vi "E710_All_VIs.vi"   [LabVIEW 2011]
uses:
  Low Level/Analog control.llb/Available Analog Commands.ctl
  Low Level/Communication.llb/Available DLL interfaces.ctl
  Low Level/Communication.llb/Available DLLs.ctl
  Low Level/Communication.llb/Available interfaces.ctl
  Low Level/Communication.llb/Termination character.ctl
  Low Level/General command.llb/Controller names.ctl
  Low Level/Analog control.llb/Global Analog.vi
  Low Level/Communication.llb/Global1.vi
  Low Level/Communication.llb/Global DaisyChain.vi
  Low Level/General command.llb/Global2 (Array).vi
  Low Level/Support.llb/Unbunde/bundle interface clusters for PI Terminal.vi
panel:
  # "E-710 PI GCS LabVIEW driver set"
  # "This VI contains all high level and low level VIs valid for E-710. See diagram for a survey of all E-710 high level\nand low level VIs. Menu / Browse / Show VI Hierarchy will show the file paths of the VIs. Global Variables \nare shown as Control as well as Indicator."
types:
  T1 = typedef "Controller names.ctl" = enum16{"None", "Analog", "C-702", "C-843", "C-843.PM", "C-844", "C-848", "C-865", "C-866", "C-867", "C-880", "E-516", "E-517", "E-709", "E-710", "E-712", "E-725", "E-753", "E-755", "E-761", "E-816", "E-861", "F-206", "M-840", "M-850", "M-8X0", "Mercury", "Mercury_GCS"}
  T2 = typedef "Termination character.ctl" = enum16{"LF", "CR", "LFCR", "CRLF"}
  T3 = typedef "Available interfaces.ctl" = u16
  T4 = typedef "Available DLLs.ctl" = u16
  T5 = typedef "Available DLL interfaces.ctl" = u16
  T6 = typedef "Available Analog Commands.ctl" = enum16{"INITIALIZE", "VOL?", "VOL ", "CLOSE", "MOV", "POS?", "VCO", "VCO?", "WAIT_WF", "TMN?", "TMX?", "VEL", "VEL?", "SAI?", "MVR", "ERR?", "#24", "STP", "*IDN?", "#5", "STE", "DRR?", "W_Wave", "HLP?", "W/R_Wave"}
  T7 = cluster{"Conversion factor":dbl[], "Velocity":dbl[], "Velocity control mode":bool, "AO.Resolution":dbl, "Lower voltage limit (V)":dbl, "Upper voltage limit (V)":dbl, "AO_WF_T (s)":dbl, "AI Sample Rate":dbl, "AI Samples/Channel":i32, "Hyperbit":bool, "Offset (V)":dbl[], "Hyperbit StayOnPos":bool, "Gain (V)":dbl[], "Bit rate (Hz)":dbl, "PWM rate (Hz)":dbl, "HyperBit Password":string, "AO.MaxRate":dbl, "Conversion offset":dbl[]}[]
  T8 = cluster{"No. of devices":i32, "Port ID":i32, "Devices":string[], "Description":string}[]
  T9 = cluster{"Conn. axes":string[], "Controller name":T1}[]
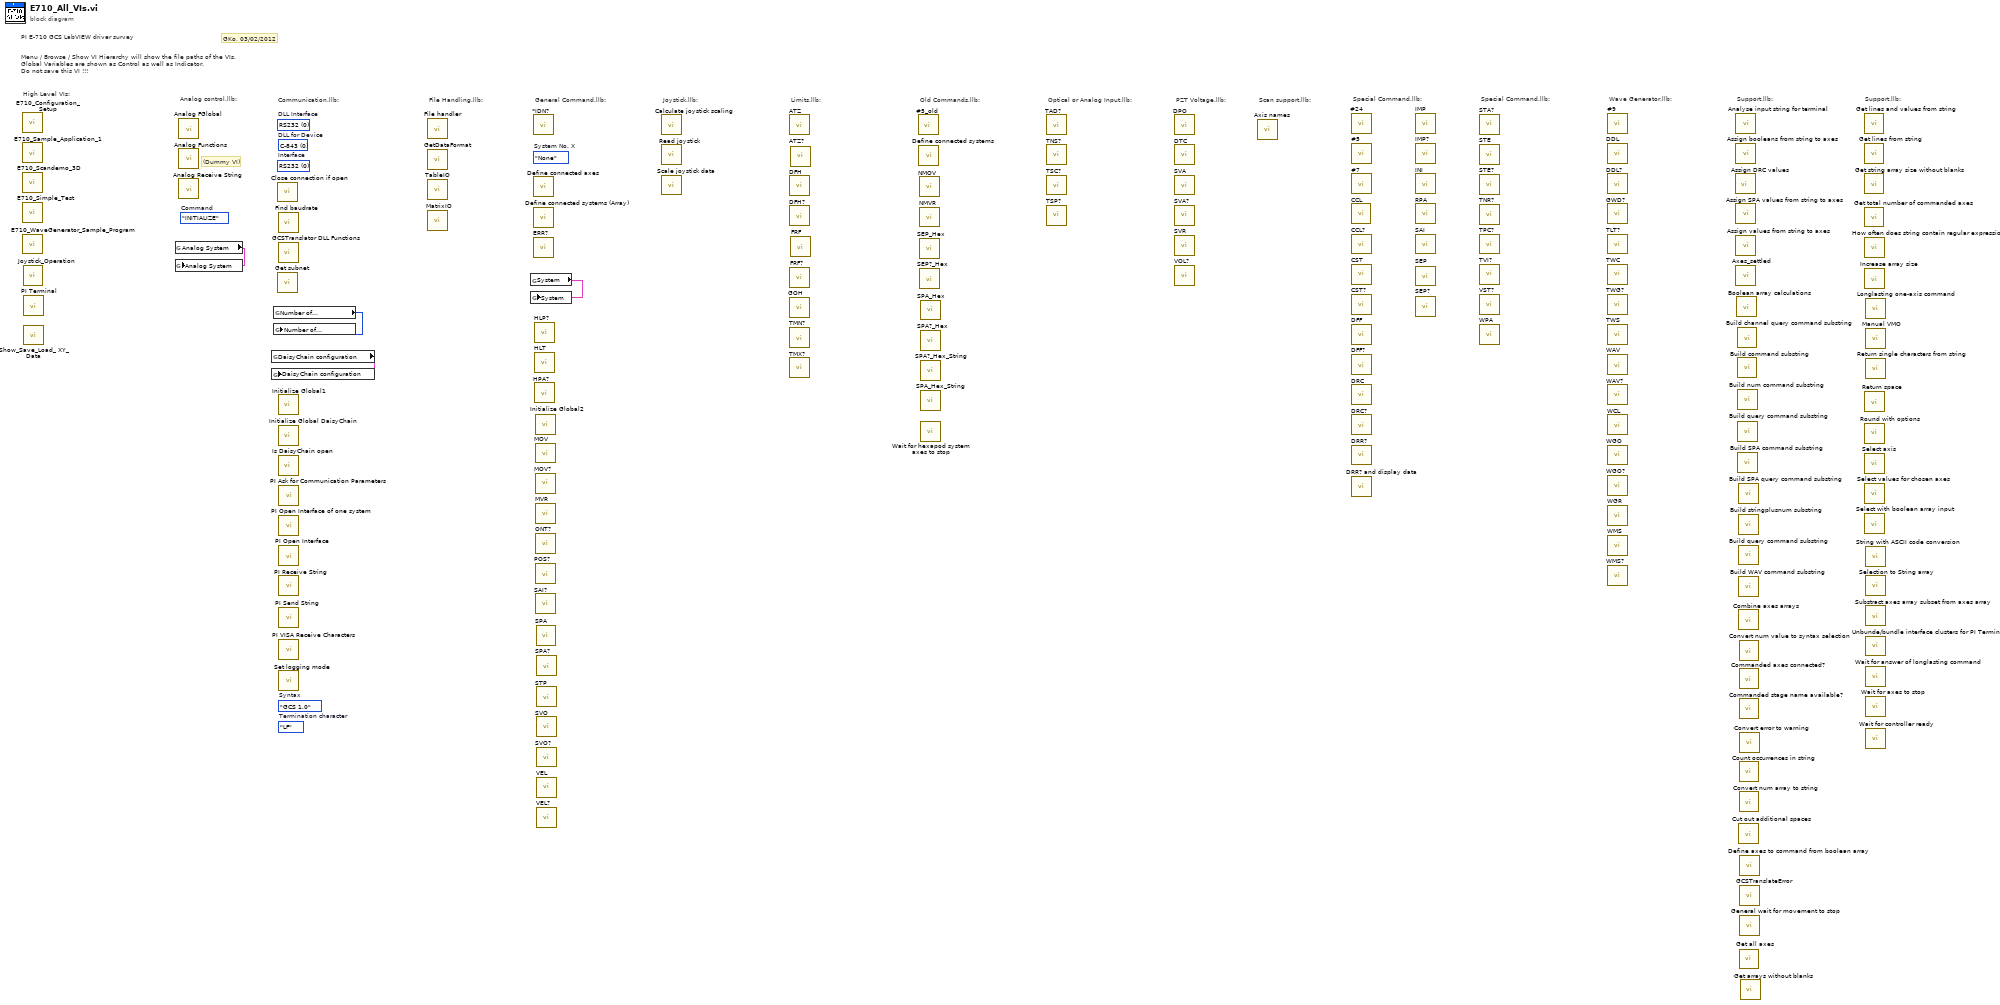
[diagram p0: block diagram]
diagram:
  (unwired) Controller_names."None"  # System No. X
  (unwired) Termination_character."LF"  # Termination character
  (unwired) enum16{"GCS 1.0", "GCS 2.0"}."GCS 1.0"  # Syntax
  (unwired) T3 0 items=["RS232", "GPIB", "DLL", "TCP-IP"]  # Interface
  (unwired) T4 0 items=["C-843", "C-844", "E-710", "C-843.PM", "C-865", "E-761", "Mercury"]  # DLL for Device
  (unwired) T5 0 items=["RS232", "GPIB", "Board", "TCP-IP", "USB"]  # DLL Interface
  (unwired) Available_Analog_Commands."INITIALIZE"  # Command
  # "Scan support.llb:"
  # "File Handling.llb:"
  # "GKo, 03/02/2012"
  # "High Level VIs:"
  # "(Dummy VI)"
  # "Analog control.llb:"
  # "Support.llb:"
  # "Wave Generator.llb:"
  # "Special Command.llb:"
  # "Support.llb:"
  # "Special Command.llb:"
  # "PZT Voltage.llb:"
  # "Optical or Analog Input.llb:"
  # "Old Commands.llb:"
  # "Limits.llb:"
  # "Joystick.llb:"
  # "General Command.llb:"
  # "Menu / Browse / Show VI Hierarchy will show the file paths of the VIs. \nGlobal Variables are shown as Control as well as Indicator.\nDo not save this VI !!!"
  # "PI E-710 GCS LabVIEW driver survey"
  # "Communication.llb:"
  n1 = call "E710_Configuration_Setup.vi"() -> ()  [unwired: 12 in, 8 out]
  n2 = call "E710_Sample_Application_1.vi"() -> ()  [unwired: 1 out]
  n3 = call "E710_Scandemo_3D.vi"() -> ()  [unwired: 28 out]
  n4 = call "E710_Simple_Test.vi"() -> ()  [unwired: 6 in, 14 out]
  n5 = call "E710_WaveGenerator_Sample_Program.vi"() -> ()  [unwired: 13 in, 7 out]
  n6 = call "Joystick_Operation.vi"() -> ()  [unwired: 15 in, 5 out]
  n7 = call "PI Terminal.vi"() -> ()  [unwired: 20 out]
  n8 = call "Show_Save_Load_ XY_Data.vi"() -> ()  [unwired: 7 in, 13 out]
  n9 = global read "Global Analog.vi" "Analog System"() -> (w4:T7)
  n10 = global write "Global Analog.vi" "Analog System"(w4) -> ()
  n11 = call "Analog FGlobal.vi"() -> ()  [unwired: 3 in, 17 out]
  n12 = call "Analog Functions.vi"() -> ()  [unwired: 7 in, 13 out]
  n13 = call "Analog Receive String.vi"() -> ()  [unwired: 5 in, 15 out]
  n14 = global read "Global DaisyChain.vi" "DaisyChain configuration"() -> (w2:T8)
  n15 = global write "Global DaisyChain.vi" "DaisyChain configuration"(w2) -> ()
  n16 = global read "Global1.vi" "Number of\nsystems"() -> (w3:i32)
  n17 = global write "Global1.vi" "Number of\nsystems"(w3) -> ()
  n18 = call "Close connection if open.vi"() -> ()  [unwired: 3 in, 17 out]
  n19 = call "Get subnet.vi"() -> ()  [unwired: 20 out]
  n20 = call "Find baudrate.vi"() -> ()  [unwired: 10 in, 10 out]
  n21 = call "GCSTranslator DLL Functions.vi"() -> ()  [unwired: 7 in, 13 out]
  n22 = call "Initialize Global1.vi"() -> ()  [unwired: 2 in, 18 out]
  n23 = call "Initialize Global DaisyChain.vi"() -> ()  [unwired: 2 in, 18 out]
  n24 = call "Is DaisyChain open.vi"() -> ()  [unwired: 2 in, 18 out]
  n25 = call "PI Ask for Communication Parameters.vi"() -> ()  [unwired: 20 out]
  n26 = call "PI Open Interface of one system.vi"() -> ()  [unwired: 12 in, 8 out]
  n27 = call "PI Open Interface.vi"() -> ()  [unwired: 12 in, 8 out]
  n28 = call "PI Receive String.vi"() -> ()  [unwired: 3 in, 17 out]
  n29 = call "PI Send String.vi"() -> ()  [unwired: 4 in, 16 out]
  n30 = call "PI VISA Receive Characters.vi"() -> ()  [unwired: 3 in, 17 out]
  n31 = call "Set logging mode.vi"() -> ()  [unwired: 4 in, 16 out]
  n32 = call "File handler.vi"() -> ()  [unwired: 6 in, 14 out]
  n33 = call "GetDataFormat.vi"() -> ()  [unwired: 2 in, 18 out]
  n34 = call "TableIO.vi"() -> ()  [unwired: 6 in, 14 out]
  n35 = call "MatrixIO.vi"() -> ()  [unwired: 7 in, 13 out]
  n36 = global read "Global2 (Array).vi" "System"() -> (w1:T9)
  n37 = global write "Global2 (Array).vi" "System"(w1) -> ()
  n38 = call "*IDN?.vi"() -> ()  [unwired: 2 in, 18 out]
  n39 = call "Define connected axes.vi"() -> ()  [unwired: 5 in, 15 out]
  n40 = call "Define connected systems (Array).vi"() -> ()  [unwired: 4 in, 16 out]
  n41 = call "ERR?.vi"() -> ()  [unwired: 2 in, 18 out]
  n42 = call "HLP?.vi"() -> ()  [unwired: 2 in, 18 out]
  n43 = call "HLT.vi"() -> ()  [unwired: 5 in, 15 out]
  n44 = call "HPA?.vi"() -> ()  [unwired: 2 in, 18 out]
  n45 = call "Initialize Global2.vi"() -> ()  [unwired: 2 in, 18 out]
  n46 = call "MOV.vi"() -> ()  [unwired: 5 in, 15 out]
  n47 = call "MOV?.vi"() -> ()  [unwired: 5 in, 15 out]
  n48 = call "MVR.vi"() -> ()  [unwired: 5 in, 15 out]
  n49 = call "ONT?.vi"() -> ()  [unwired: 5 in, 15 out]
  n50 = call "POS?.vi"() -> ()  [unwired: 5 in, 15 out]
  n51 = call "SAI?.vi"() -> ()  [unwired: 5 in, 15 out]
  n52 = call "SPA.vi"() -> ()  [unwired: 10 in, 10 out]
  n53 = call "SPA?.vi"() -> ()  [unwired: 7 in, 13 out]
  n54 = call "STP.vi"() -> ()  [unwired: 5 in, 15 out]
  n55 = call "SVO.vi"() -> ()  [unwired: 5 in, 15 out]
  n56 = call "SVO?.vi"() -> ()  [unwired: 5 in, 15 out]
  n57 = call "VEL.vi"() -> ()  [unwired: 6 in, 14 out]
  n58 = call "VEL?.vi"() -> ()  [unwired: 5 in, 15 out]
  n59 = call "Calculate joystick scaling.vi"() -> ()  [unwired: 6 in, 14 out]
  n60 = call "Read joystick.vi"() -> ()  [unwired: 2 in, 18 out]
  n61 = call "Scale joystick data.vi"() -> ()  [unwired: 8 in, 12 out]
  n62 = call "ATZ.vi"() -> ()  [unwired: 6 in, 14 out]
  n63 = call "DFH.vi"() -> ()  [unwired: 5 in, 15 out]
  n64 = call "DFH?.vi"() -> ()  [unwired: 5 in, 15 out]
  n65 = call "FRF?.vi"() -> ()  [unwired: 5 in, 15 out]
  n66 = call "GOH.vi"() -> ()  [unwired: 5 in, 15 out]
  n67 = call "TMN?.vi"() -> ()  [unwired: 5 in, 15 out]
  n68 = call "TMX?.vi"() -> ()  [unwired: 5 in, 15 out]
  n69 = call "ATZ?.vi"() -> ()  [unwired: 5 in, 15 out]
  n70 = call "FRF.vi"() -> ()  [unwired: 5 in, 15 out]
  n71 = call "#5_old.vi"() -> ()  [unwired: 2 in, 18 out]
  n72 = call "Define connected systems.vi"() -> ()  [unwired: 4 in, 16 out]
  n73 = call "NMOV.vi"() -> ()  [unwired: 5 in, 15 out]
  n74 = call "NMVR.vi"() -> ()  [unwired: 5 in, 15 out]
  n75 = call "SEP_Hex.vi"() -> ()  [unwired: 6 in, 14 out]
  n76 = call "SEP?_Hex.vi"() -> ()  [unwired: 5 in, 15 out]
  n77 = call "SPA_Hex.vi"() -> ()  [unwired: 6 in, 14 out]
  n78 = call "SPA?_Hex.vi"() -> ()  [unwired: 5 in, 15 out]
  n79 = call "SPA?_Hex_String.vi"() -> ()  [unwired: 5 in, 15 out]
  n80 = call "SPA_Hex_String.vi"() -> ()  [unwired: 5 in, 15 out]
  n81 = call "Wait for hexapod system axes to stop.vi"() -> ()  [unwired: 5 in, 15 out]
  n82 = call "TAD?.vi"() -> ()  [unwired: 5 in, 15 out]
  n83 = call "TNS?.vi"() -> ()  [unwired: 5 in, 15 out]
  n84 = call "TSC?.vi"() -> ()  [unwired: 2 in, 18 out]
  n85 = call "TSP?.vi"() -> ()  [unwired: 5 in, 15 out]
  n86 = call "DPO.vi"() -> ()  [unwired: 5 in, 15 out]
  n87 = call "DTC.vi"() -> ()  [unwired: 4 in, 16 out]
  n88 = call "SVA.vi"() -> ()  [unwired: 5 in, 15 out]
  n89 = call "SVA?.vi"() -> ()  [unwired: 5 in, 15 out]
  n90 = call "SVR.vi"() -> ()  [unwired: 5 in, 15 out]
  n91 = call "VOL?.vi"() -> ()  [unwired: 5 in, 15 out]
  n92 = call "Axis names.vi"() -> ()  [unwired: 1 in, 19 out]
  n93 = call "CCL.vi"() -> ()  [unwired: 4 in, 16 out]
  n94 = call "#24.vi"() -> ()  [unwired: 2 in, 18 out]
  n95 = call "#5.vi"() -> ()  [unwired: 2 in, 18 out]
  n96 = call "#7.vi"() -> ()  [unwired: 2 in, 18 out]
  n97 = call "CCL?.vi"() -> ()  [unwired: 2 in, 18 out]
  n98 = call "CST.vi"() -> ()  [unwired: 4 in, 16 out]
  n99 = call "CST?.vi"() -> ()  [unwired: 5 in, 15 out]
  n100 = call "DFF.vi"() -> ()  [unwired: 5 in, 15 out]
  n101 = call "DFF?.vi"() -> ()  [unwired: 5 in, 15 out]
  n102 = call "DRC.vi"() -> ()  [unwired: 6 in, 14 out]
  n103 = call "DRC?.vi"() -> ()  [unwired: 4 in, 16 out]
  n104 = call "DRR?.vi"() -> ()  [unwired: 7 in, 13 out]
  n105 = call "DRR? and display data.vi"() -> ()  [unwired: 7 in, 13 out]
  n106 = call "IMP.vi"() -> ()  [unwired: 5 in, 15 out]
  n107 = call "IMP?.vi"() -> ()  [unwired: 6 in, 14 out]
  n108 = call "INI.vi"() -> ()  [unwired: 5 in, 15 out]
  n109 = call "RPA.vi"() -> ()  [unwired: 6 in, 14 out]
  n110 = call "SAI.vi"() -> ()  [unwired: 4 in, 16 out]
  n111 = call "SEP.vi"() -> ()  [unwired: 11 in, 9 out]
  n112 = call "SEP?.vi"() -> ()  [unwired: 7 in, 13 out]
  n113 = call "STA?.vi"() -> ()  [unwired: 5 in, 15 out]
  n114 = call "STE.vi"() -> ()  [unwired: 6 in, 14 out]
  n115 = call "STE?.vi"() -> ()  [unwired: 6 in, 14 out]
  n116 = call "TNR?.vi"() -> ()  [unwired: 2 in, 18 out]
  n117 = call "TPC?.vi"() -> ()  [unwired: 2 in, 18 out]
  n118 = call "TVI?.vi"() -> ()  [unwired: 3 in, 17 out]
  n119 = call "VST?.vi"() -> ()  [unwired: 2 in, 18 out]
  n120 = call "WPA.vi"() -> ()  [unwired: 7 in, 13 out]
  n121 = call "#9.vi"() -> ()  [unwired: 2 in, 18 out]
  n122 = call "DDL.vi"() -> ()  [unwired: 6 in, 14 out]
  n123 = call "DDL?.vi"() -> ()  [unwired: 5 in, 15 out]
  n124 = call "GWD?.vi"() -> ()  [unwired: 6 in, 14 out]
  n125 = call "TLT?.vi"() -> ()  [unwired: 2 in, 18 out]
  n126 = call "TWC.vi"() -> ()  [unwired: 2 in, 18 out]
  n127 = call "TWG?.vi"() -> ()  [unwired: 2 in, 18 out]
  n128 = call "TWS.vi"() -> ()  [unwired: 5 in, 15 out]
  n129 = call "WAV.vi"() -> ()  [unwired: 18 in, 10 out]
  n130 = call "WAV?.vi"() -> ()  [unwired: 4 in, 16 out]
  n131 = call "WCL.vi"() -> ()  [unwired: 5 in, 15 out]
  n132 = call "WGO.vi"() -> ()  [unwired: 4 in, 16 out]
  n133 = call "WGO?.vi"() -> ()  [unwired: 5 in, 15 out]
  n134 = call "WGR.vi"() -> ()  [unwired: 2 in, 18 out]
  n135 = call "WMS.vi"() -> ()  [unwired: 5 in, 15 out]
  n136 = call "WMS?.vi"() -> ()  [unwired: 5 in, 15 out]
  n137 = call "Assign DRC values.vi"() -> ()  [unwired: 3 in, 17 out]
  n138 = call "Analyse input string for terminal.vi"() -> ()  [unwired: 2 in, 18 out]
  n139 = call "Assign booleans from string to axes.vi"() -> ()  [unwired: 5 in, 15 out]
  n140 = call "Assign SPA values from string to axes.vi"() -> ()  [unwired: 7 in, 13 out]
  n141 = call "Assign values from string to axes.vi"() -> ()  [unwired: 6 in, 14 out]
  n142 = call "Axes_settled.vi"() -> ()  [unwired: 5 in, 15 out]
  n143 = call "Boolean array calculations.vi"() -> ()  [unwired: 4 in, 16 out]
  n144 = call "Build channel query command substring.vi"() -> ()  [unwired: 7 in, 13 out]
  n145 = call "Build command substring.vi"() -> ()  [unwired: 7 in, 13 out]
  n146 = call "Build num command substring.vi"() -> ()  [unwired: 3 in, 17 out]
  n147 = call "Build query command substring.vi"() -> ()  [unwired: 5 in, 15 out]
  n148 = call "Build SPA command substring.vi"() -> ()  [unwired: 10 in, 10 out]
  n149 = call "Build SPA query command substring.vi"() -> ()  [unwired: 5 in, 15 out]
  n150 = call "Build stringplusnum substring.vi"() -> ()  [unwired: 10 in, 10 out]
  n151 = call "Build query command substring.vi"() -> ()  [unwired: 5 in, 15 out]
  n152 = call "Build WAV command substring.vi"() -> ()  [unwired: 16 in, 12 out]
  n153 = call "Combine axes arrays.vi"() -> ()  [unwired: 2 in, 18 out]
  n154 = call "Cut out additional spaces.vi"() -> ()  [unwired: 2 in, 18 out]
  n155 = call "Convert num value to syntax selection.vi"() -> ()  [unwired: 1 in, 19 out]
  n156 = call "Commanded axes connected?.vi"() -> ()  [unwired: 3 in, 17 out]
  n157 = call "Commanded stage name available?.vi"() -> ()  [unwired: 3 in, 17 out]
  n158 = call "Count occurrences in string.vi"() -> ()  [unwired: 2 in, 18 out]
  n159 = call "Convert num array to string.vi"() -> ()  [unwired: 2 in, 18 out]
  n160 = call "Get all axes.vi"() -> ()  [unwired: 1 in, 19 out]
  n161 = call "Convert error to warning.vi"() -> ()  [unwired: 2 in, 18 out]
  n162 = call "Define axes to command from boolean array.vi"() -> ()  [unwired: 4 in, 16 out]
  n163 = call "GCSTranslateError.vi"() -> ()  [unwired: 1 in, 19 out]
  n164 = call "General wait for movement to stop.vi"() -> ()  [unwired: 8 in, 12 out]
  n165 = call "Get arrays without blanks.vi"() -> ()  [unwired: 3 in, 17 out]
  n166 = call "Get lines and values from string.vi"() -> ()  [unwired: 2 in, 18 out]
  n167 = call "Get lines from string.vi"() -> ()  [unwired: 3 in, 17 out]
  n168 = call "Get string array size without blanks.vi"() -> ()  [unwired: 1 in, 19 out]
  n169 = call "Get total number of commanded axes.vi"() -> ()  [unwired: 2 in, 18 out]
  n170 = call "How often does string contain regular expression?.vi"() -> ()  [unwired: 2 in, 18 out]
  n171 = call "Increase array size.vi"() -> ()  [unwired: 3 in, 17 out]
  n172 = call "Return space.vi"() -> ()  [unwired: 2 in, 18 out]
  n173 = call "Round with options.vi"() -> ()  [unwired: 4 in, 16 out]
  n174 = call "Select axis.vi"() -> ()  [unwired: 2 in, 18 out]
  n175 = call "Select values for chosen axes.vi"() -> ()  [unwired: 5 in, 15 out]
  n176 = call "Select with boolean array input.vi"() -> ()  [unwired: 4 in, 16 out]
  n177 = call "Longlasting one-axis command.vi"() -> ()  [unwired: 7 in, 13 out]
  n178 = call "Manual VMO.vi"() -> ()  [unwired: 6 in, 14 out]
  n179 = call "Return single characters from string.vi"() -> ()  [unwired: 3 in, 17 out]
  n180 = call "String with ASCII code conversion.vi"() -> ()  [unwired: 1 in, 19 out]
  n181 = call "Selection to String array.vi"() -> ()  [unwired: 2 in, 18 out]
  n182 = call "Substract axes array subset from axes array.vi"() -> ()  [unwired: 2 in, 18 out]
  n183 = call "Unbunde/bundle interface clusters for PI Terminal.vi"() -> ()  [unwired: 6 in, 14 out]
  n184 = call "Wait for answer of longlasting command.vi"() -> ()  [unwired: 3 in, 17 out]
  n185 = call "Wait for axes to stop.vi"() -> ()  [unwired: 7 in, 13 out]
  n186 = call "Wait for controller ready.vi"() -> ()  [unwired: 4 in, 16 out]
